vi "Read send from port.vi"(8 "error in (no error)":errorcluster, 11 "TEC configuration in":refnum<class "TEC configuration.lvclass">) -> (0 "error out":errorcluster, 2 "send from port":u16=61556, 3 "TEC configuration out":refnum<class "TEC configuration.lvclass">)   [LabVIEW 2013, in "TEC configuration.lvclass"]
uses:
  TEC configuration.lvclass
  TEC configuration.lvclass/TEC configuration.ctl
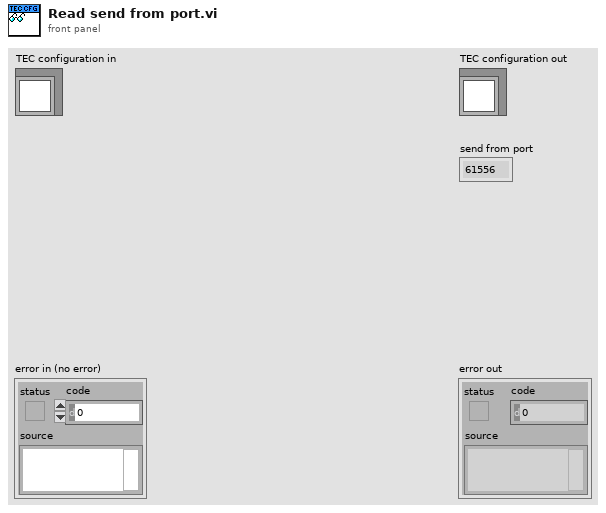
[diagram p1: front panel]
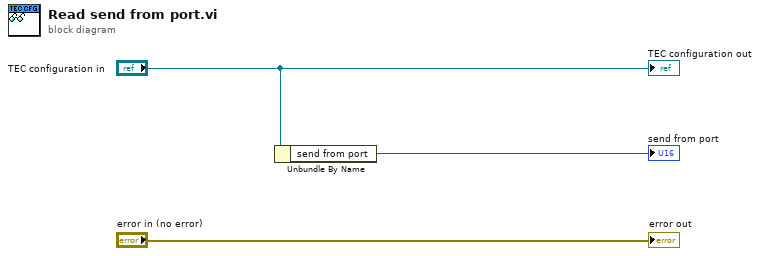
[diagram p0: block diagram]
diagram:
  n1 = Unbundle By Name("TEC configuration in") -> ("send from port"=→"send from port":u16)
  "error out" <- "error in (no error)"
  "TEC configuration out" <- "TEC configuration in"
